vi "Main.vi"() -> ()   [LabVIEW 2013]
uses:
  <vilib>/myRIO/Common/Instrument Driver Framework/myRIO v1.0/DIO/vis/myRIO v1.1 Open DIO.vi
  <vilib>/myRIO/Instrument Drivers/Onboard IO/DIO/vis/Smart Open.vi
  <vilib>/myRIO/Common/Instrument Driver Framework/myRIO v1.0/UART/vis/myRIO v1.0 Close UART.vi
  <vilib>/myRIO/Common/Instrument Driver Framework/Utilities/vis/Validate Channels.vi
  <vilib>/myRIO/Common/Instrument Driver Framework/myRIO v1.0/DIO/vis/myRIO v1.0 Reserve DIO.vi
  <vilib>/myRIO/Common/Instrument Driver Framework/myRIO v1.0/Resource Manager/vis/myRIO v1.0 Reserve Channel List.vi
  <vilib>/myRIO/Common/Instrument Driver Framework/myRIO v1.0/DIO/vis/myRIO v1.0 Build MUX Configuration DIO.vi
  <vilib>/myRIO/Common/Instrument Driver Framework/myRIO v1.0/Resource Manager/vis/myRIO v1.0 Reserve Channel.vi
  <vilib>/myRIO/Common/Instrument Driver Framework/myRIO v1.0/Resource Manager/vis/myRIO v1.0 Unreserve Channel.vi
  <vilib>/myRIO/Common/Instrument Driver Framework/myRIO v1.0/Resource Manager/vis/myRIO v1.0 Create Configuration List.vi
  <vilib>/myRIO/Common/Instrument Driver Framework/myRIO v1.0/Resource Manager/vis/myRIO v1.0 Build Mutex Name.vi
  <vilib>/myRIO/Common/Instrument Driver Framework/myRIO v1.0/myRIO v1.1 Open.vi
  <vilib>/Utility/VariantDataType/GetNumericInfo.vi
  <vilib>/Utility/error.llb/Error Cluster From Error Code.vi
  <vilib>/myRIO/Common/Instrument Driver Framework/Utilities/vis/IO Manager.vi
  <vilib>/myRIO/Common/Instrument Driver Framework/Utilities/vis/Configuration Manager.vi
  <vilib>/myRIO/Common/Instrument Driver Framework/myRIO v1.0/Resource Manager/vis/myRIO v1.0 Configure IO.vi
  <vilib>/myRIO/Common/Instrument Driver Framework/myRIO v1.0/myRIO v1.0 Close.vi
  <vilib>/myRIO/Common/Instrument Driver Framework/myRIO v1.0/DIO/vis/myRIO v1.0 Read DIO.vi
  <vilib>/myRIO/Common/Instrument Driver Framework/myRIO v1.0/DIO/vis/myRIO v1.0 Write DIO.vi
  <vilib>/myRIO/Common/Instrument Driver Framework/Utilities/vis/FPGA Ref Manager.vi
  <vilib>/myRIO/Common/Instrument Driver Framework/myRIO v1.0/myRIO v1.0 Reset FPGA.vi
  <vilib>/myRIO/Instrument Drivers/Utilities/Utilities.lvlib
  <vilib>/myRIO/Instrument Drivers/Onboard IO/DIO/DIO.lvlib
panel:
  out "Scan":bool[](array[boolean])
  out "Keypad buttons":bool[][](array[boolean])
  in  "[ESC]":bool
  # "Keypad demo"
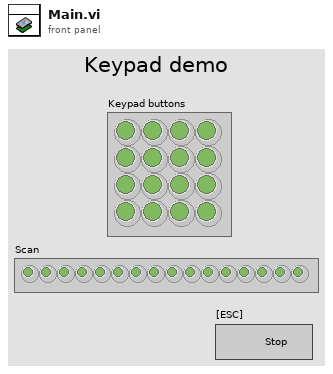
[diagram p1: front panel]
types:
  T1 = typedef "DIO.lvlib/DIO Reference.ctl" = cluster{"myRIO Reference":T2, "DIO Channels List":T6}
  T2 = typedef "myRIO Generic Hardware Reference.ctl" = cluster{"myRIO Model":T3, "myRIO Hardware Reference":T4}
  T3 = typedef "Hardware Version Enum.ctl" = enum16{"Unknown", "myRIO-1900", "myRIO-1950"}
  T4 = typedef "myRIO v1.0 Reference.ctl" = cluster{"Generic FPGA Reference":T5, "Allow multiple opens":bool}
  T5 = typedef "Generic FPGA Reference.ctl" = refnum<k20>
  T6 = typedef "DIO Channels List.ctl" = T7[]
  T7 = typedef "DIO Channels Enum.ctl" = enum16{"Not Connected", "C/DIO0", "C/DIO1", "C/DIO2", "C/DIO3", "C/DIO4", "C/DIO5", "C/DIO6", "C/DIO7", "A/DIO0", "A/DIO1", "A/DIO2", "A/DIO3", "A/DIO4", "A/DIO5", "A/DIO6", "A/DIO7", "A/DIO8", "A/DIO9", "A/DIO10", "A/DIO11", "A/DIO12", "A/DIO13", "A/DIO14", "A/DIO15", "B/DIO0", "B/DIO1", "B/DIO2", "B/DIO3", "B/DIO4", "B/DIO5", "B/DIO6", "B/DIO7", "B/DIO8", "B/DIO9", "B/DIO10", "B/DIO11", "B/DIO12", "B/DIO13", "B/DIO14", "B/DIO15", "LED0", "LED1", "LED2", "LED3", "Button0"}
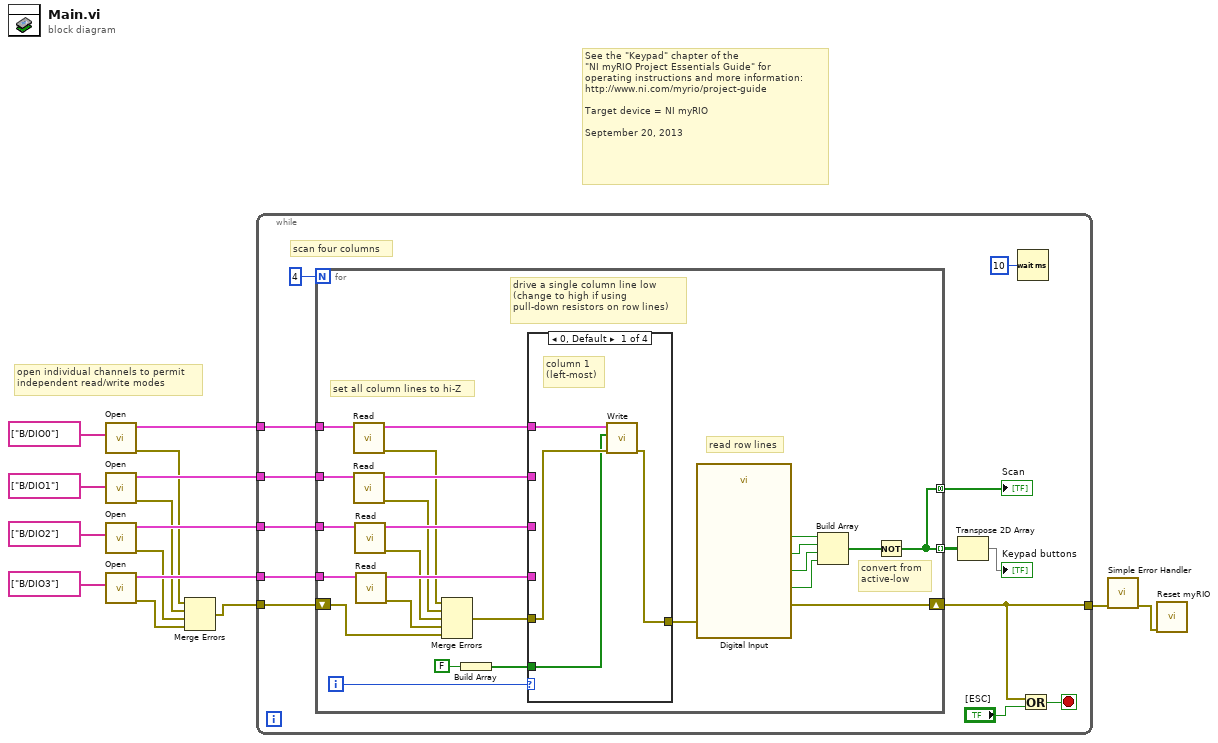
[diagram p0: block diagram]
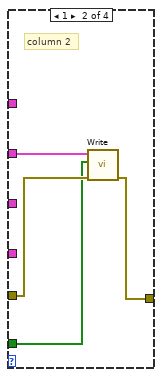
[diagram p2: hidden frame]
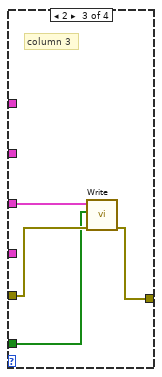
[diagram p3: hidden frame]
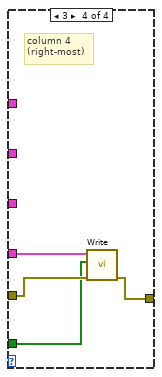
[diagram p4: hidden frame]
diagram:
  # "See the \"Keypad\" chapter of the\n\"NI myRIO Project Essentials Guide\" for\noperating instructions and more information: \nhttp://www.ni.com/myrio/project-guide\n\nTarget device = NI myRIO\n\nSeptember 20, 2013"
  # "open individual channels to permit\nindependent read/write modes"
  n1 = call <vilib>:"Open.vi"("Channel Names"=tag[] ["B/DIO0"]) -> ("error out"=w5:errorcluster, "DIO Ref Out"=w9:T1)  [unwired: 9 in]
  n2 = call <vilib>:"Open.vi"("Channel Names"=tag[] ["B/DIO1"]) -> ("error out"=w4:errorcluster, "DIO Ref Out"=w8:T1)  [unwired: 9 in]
  n3 = call <vilib>:"Open.vi"("Channel Names"=tag[] ["B/DIO2"]) -> ("error out"=w3:errorcluster, "DIO Ref Out"=w7:T1)  [unwired: 9 in]
  n4 = call <vilib>:"Open.vi"("Channel Names"=tag[] ["B/DIO3"]) -> ("error out"=w2:errorcluster, "DIO Ref Out"=w6:T1)  [unwired: 9 in]
  n5 = Merge Errors "Merge Errors"(w5, w4, w3, w2) -> (w1:errorcluster)
  n6 = while {
    tunnel: [w24] -> w15
    tunnel: w9 -> [w20]
    tunnel: w8 -> [w19]
    tunnel: w7 -> [w18]
    tunnel: w6 -> [w17]
    tunnel: w1 -> [w16]
    stop <- w28 stop-if-true
    # "scan four columns"
    n7 = for {
      N: 4 -> [_]
      tunnel: [w46] -> w23 mode=indexing
      shift-right: [w48] -> w24
      shift-left: w16 -> [w32]
      tunnel: [w46] -> w21 mode=concatenating
      tunnel: w20 -> [w45]
      tunnel: w19 -> [w42]
      tunnel: w18 -> [w43]
      tunnel: w17 -> [w44]
      i -> [w53]
      # "convert from\nactive-low"
      # "set all column lines to hi-Z"
      # "read row lines"
      # "drive a single column line low\n(change to high if using \npull-down resistors on row lines)"
      n8 = call <vilib>:"Read.vi"("DIO Ref In"=w45) -> ("error out"=w36:errorcluster, "DIO Ref Out"=w41:T1)  [unwired: 8 in, 1 out]
      n9 = call <vilib>:"Read.vi"("DIO Ref In"=w42) -> ("error out"=w35:errorcluster, "DIO Ref Out"=w40:T1)  [unwired: 8 in, 1 out]
      n10 = call <vilib>:"Read.vi"("DIO Ref In"=w43) -> ("error out"=w34:errorcluster, "DIO Ref Out"=w39:T1)  [unwired: 8 in, 1 out]
      n11 = call <vilib>:"Read.vi"("DIO Ref In"=w44) -> ("error out"=w33:errorcluster, "DIO Ref Out"=w38:T1)  [unwired: 8 in, 1 out]
      n12 = Merge Errors(w36, w35, w34, w33, w32) -> (w31:errorcluster)
      n13 = Build Array "Build Array"(FALSE) -> (w29:bool[])
      n14 = case shown="0, Default" w53 {
        tunnel: w41 -> [w57 _ _ _]
        tunnel: w40 -> [_ w61 _ _]
        tunnel: w39 -> [_ _ w65 _]
        tunnel: w38 -> [_ _ _ w69]
        tunnel: [w56 w60 w64 w68] -> w37
        tunnel: w31 -> [w55 w59 w63 w67]
        tunnel: w29 -> [w54 w58 w62 w66]
        frame 0, Default {
          # "column 1\n(left-most)"
          n15 = call <vilib>:"Write.vi"("error in (no error)"=w55, "Values"=w54, "DIO Ref In"=w57) -> ("error out"=w56:errorcluster)  [unwired: 6 in, 1 out]
        }
        frame 1 {
          # "column 2"
          n16 = call <vilib>:"Write.vi"("error in (no error)"=w59, "Values"=w58, "DIO Ref In"=w61) -> ("error out"=w60:errorcluster)  [unwired: 6 in, 1 out]
        }
        frame 2 {
          # "column 3"
          n17 = call <vilib>:"Write.vi"("error in (no error)"=w63, "Values"=w62, "DIO Ref In"=w65) -> ("error out"=w64:errorcluster)  [unwired: 6 in, 1 out]
        }
        frame 3 {
          # "column 4\n(right-most)"
          n18 = call <vilib>:"Write.vi"("error in (no error)"=w67, "Values"=w66, "DIO Ref In"=w69) -> ("error out"=w68:errorcluster)  [unwired: 6 in, 1 out]
        }
      }
      n19 = call "Digital Input"("error in (no error)"=w37) -> ("B/DIO4 (Pin 19)"=w52:bool, "B/DIO5 (Pin 21)"=w51:bool, "B/DIO6 (Pin 23)"=w50:bool, "B/DIO7 (Pin 25)"=w49:bool, "error out"=w48:errorcluster)  [unwired: 22 in]
      n20 = Build Array "Build Array"(w52, w51, w50, w49) -> (w47:bool[])
      n21 = Not(x=w47) -> (.not. x?=w46:bool[])
    }
    "Scan" <- w21
    n22 = Transpose 2D Array(2D array=w23) -> (transposed array=→"Keypad buttons":bool[][])
    n23 = Wait (ms)(milliseconds to wait=u32 10) -> ()  [unwired: 1 out]
    n24 = Or(x=w24, y="[ESC]") -> (x .or. y?=w28:bool)
  }
  n25 = call <vilib>:"Simple Error Handler.vi"("error in (no error)"=w15) -> ("error out"=w14:errorcluster)  [unwired: 4 in, 4 out]
  n26 = call <vilib>:"Reset myRIO.vi"("error in (no error)"=w14) -> ()  [unwired: 10 in, 1 out]
